vi "Get Shared Data Dir.vi"() -> (0 "Error Out":errorcluster, 3 "Data Directory Path":path)   [LabVIEW 2018]
doc: "Returns path to a shared data directory on all platforms. Creates intermediate directories if necessary with read/write access\nScott Hannahs <sth@magnet.fsu.edu>\nAuthor: Scott Hannahs <sth@magnet.fsu.edu>\nCopyright 2018 Florida State University, All rights reserved."
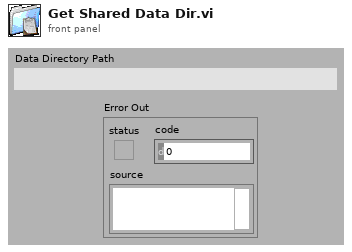
[diagram p1: front panel]
types:
  T1 = enum16{"CSIDL_DESKTOP", "CSIDL_INTERNET", "CSIDL_PROGRAMS", "CSIDL_CONTROLS", "CSIDL_PRINTERS\n", "CSIDL_PERSONAL", "CSIDL_FAVORITES", "CSIDL_STARTUP", "CSIDL_RECENT", "CSIDL_SENDTO", "CSIDL_BITBUCKET", "CSIDL_STARTMENU", "DUMMY1", "DUMMY2", "DUMMY3", "DUMMY4", "CSIDL_DESKTOPDIRECTORY", "CSIDL_DRIVES", "CSIDL_NETWORK", "CSIDL_NETHOOD", "CSIDL_FONTS", "CSIDL_TEMPLATES", "CSIDL_COMMON_STARTMENU", "CSIDL_COMMON_PROGRAMS", "CSIDL_COMMON_STARTUP", "CSIDL_COMMON_DESKTOPDIRECTORY", "CSIDL_APPDATA", "CSIDL_PRINTHOOD", "CSIDL_LOCAL_APPDATA", "CSIDL_ALTSTARTUP", "CSIDL_COMMON_ALTSTARTUP", "CSIDL_COMMON_FAVORITES", "CSIDL_INTERNET_CACHE", "CSIDL_COOKIES", "CSIDL_HISTORY", "CSIDL_COMMON_APPDATA", "CSIDL_WINDOWS", "CSIDL_SYSTEM", "CSIDL_PROGRAM_FILES", "CSIDL_MYPICTURES", "CSIDL_PROFILE", "CSIDL_SYSTEMX86", "CSIDL_PROGRAM_FILESX86", "CSIDL_PROGRAM_FILES_COMMON", "CSIDL_PROGRAM_FILES_COMMONX86", "CSIDL_COMMON_TEMPLATES", "CSIDL_COMMON_DOCUMENTS", "CSIDL_COMMON_ADMINTOOLS", "CSIDL_ADMINTOOLS"}
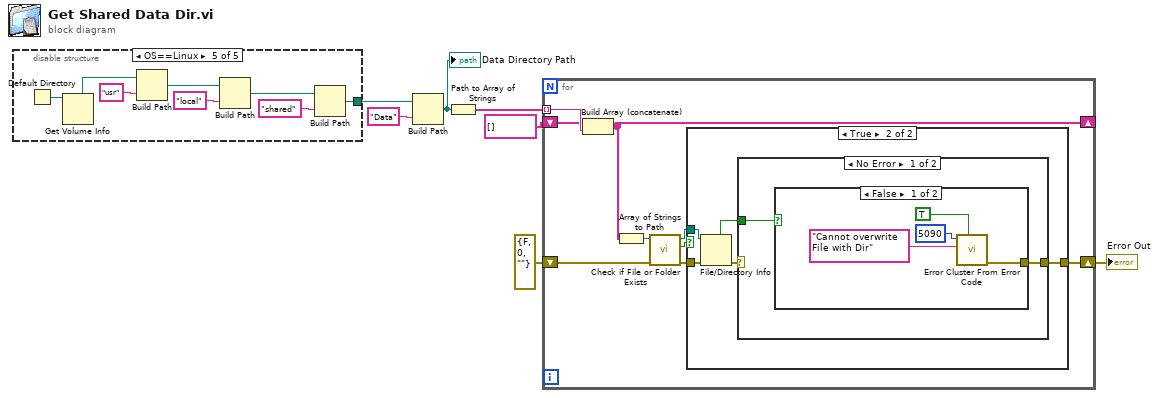
[diagram p0: block diagram]
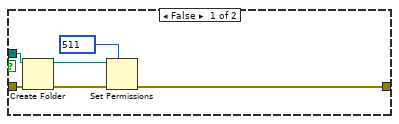
[diagram p2: hidden frame]
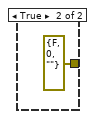
[diagram p3: hidden frame]
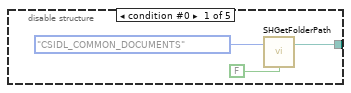
[diagram p5: hidden frame]
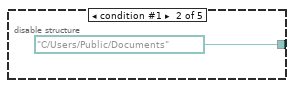
[diagram p6: hidden frame]
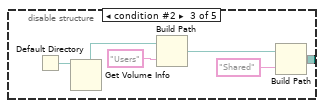
[diagram p7: hidden frame]
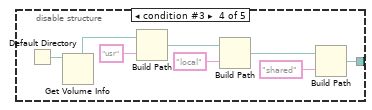
[diagram p8: hidden frame]
diagram:
  n1 = disable-structure shown="OS==Linux" {
    disable-tunnel: [w8 path "C:/Users/Public/Documents" ("Path") w12 w20 w28] -> w4
    frame condition #0 {
      n2 = call "SHGetFolderPath.vi"("Return Current Path:F / Default Path:T (F)"=FALSE, "CSIDL"=T1."CSIDL_COMMON_DOCUMENTS") -> ("Path"=w8:path)  [unwired: 2 in, 1 out]
    }
    frame condition #1 {
    }
    frame condition #2 {
      n3 = Default Directory() -> (w14:path)
      n4 = Get Volume Info(11:w14) -> (5:w13:path)  [unwired: 1 in, 5 out]
      n5 = Build Path(base path=w13, name or relative path="Users") -> (appended path=w15:path)
      n6 = Build Path(base path=w15, name or relative path="Shared") -> (appended path=w12:path)
    }
    frame condition #3 {
      n7 = Default Directory() -> (w18:path)
      n8 = Get Volume Info(11:w18) -> (5:w22:path)  [unwired: 1 in, 5 out]
      n9 = Build Path(base path=w22, name or relative path="usr") -> (appended path=w23:path)
      n10 = Build Path(base path=w23, name or relative path="local") -> (appended path=w21:path)
      n11 = Build Path(base path=w21, name or relative path="shared") -> (appended path=w20:path)
    }
    frame condition #4 (active) {
      n12 = Default Directory() -> (w26:path)
      n13 = Get Volume Info(11:w26) -> (5:w30:path)  [unwired: 1 in, 5 out]
      n14 = Build Path(base path=w30, name or relative path="usr") -> (appended path=w31:path)
      n15 = Build Path(base path=w31, name or relative path="local") -> (appended path=w29:path)
      n16 = Build Path(base path=w29, name or relative path="shared") -> (appended path=w28:path)
    }
  }
  n17 = Build Path(base path=w4, name or relative path="Data") -> (appended path=w2:path)
  "Data Directory Path" <- w2
  n18 = Path to Array of Strings(0:w2) -> (2:w7:string[])  [unwired: 1 out]
  n19 = for {
    tunnel: w7 -> [w42] mode=indexing
    shift-right: [w40] -> _
    shift-left: string[] [] -> [w41]
    shift-right: [w34] -> w3
    shift-left: errorcluster {"status"=FALSE, "code"=0, "source"=""} ("error IO") -> [w35]
    n20 = Build Array (concatenate)(w41, w42) -> (w40:string[])
    n21 = Array of Strings to Path(0:w40) -> (2:w39:path)  [unwired: 1 in]
    n22 = call <vilib>:"Check if File or Folder Exists.vi"("error in (no error)"=w35, "path"=w39) -> ("error out"=w36:errorcluster, "file or folder exists?"=w38:bool, "dup path"=w37:path)  [unwired: 7 in]
    n23 = case shown="True" w38 {
      tunnel: w37 -> [w48 w52]
      tunnel: w36 -> [w47 w53]
      tunnel: [w43 w50] -> w34
      frame False {
        n24 = Create Folder(path (use dialog)=w48, error in=w47) -> (created path=w46:path, error out=w45:errorcluster)  [unwired: 1 in, 1 out]
        n25 = Set Permissions(7:i16 511 ("permissions"), 8:w45, 11:w46) -> (0:w43:errorcluster)  [unwired: 2 in, 1 out]
      }
      frame True {
        n26 = File/Directory Info(path=w52, error in=w53) -> (directory=w49:bool, error out=w51:errorcluster)  [unwired: 5 out]
        n27 = case shown="No Error" w51 {
          selector: w51 -> [_ w61]
          tunnel: [w55 w61] -> w50
          tunnel: w49 -> [w54 _]
          frame No Error {
            n28 = case shown="False" w54 {
              tunnel: [w56 errorcluster {"status"=FALSE, "code"=0, "source"=""} ("error out")] -> w55
              frame False {
                n29 = call <vilib>:"Error Cluster From Error Code.vi"("show call chain? (False)"=TRUE, "error message (\"\")"="Cannot overwrite File with Dir" ("error message (\"\")"), "error code (0)"=5090 ("code")) -> ("error out"=w56:errorcluster)  [unwired: 6 in]
              }
              frame True {
              }
            }
          }
          frame Error {
          }
        }
      }
    }
  }
  "Error Out" <- w3
